vi "aux-builder.parser.vi"(8 "error in":errorcluster, 10 "Proc Name":string, 11 "Flow":T2[](array[typedef])) -> (0 "error out":errorcluster, 3 "Aux Conf out":T1={"Source"="Source ...", "SourceStatus"=FALSE, "Dest"="Auxiliary ...", "DestStatus"=FALSE, "Pulse"=0, "Period"=0, "Proc Name"=""} {"Period" format="Period [s]: %d"; "Pulse" format="Pulse [s]: %d"})   [LabVIEW 2024]
uses:
  controls/UiStepBuilder.ctl
  controls/type.step-builder.ctl
  controls/type.aux.ctl
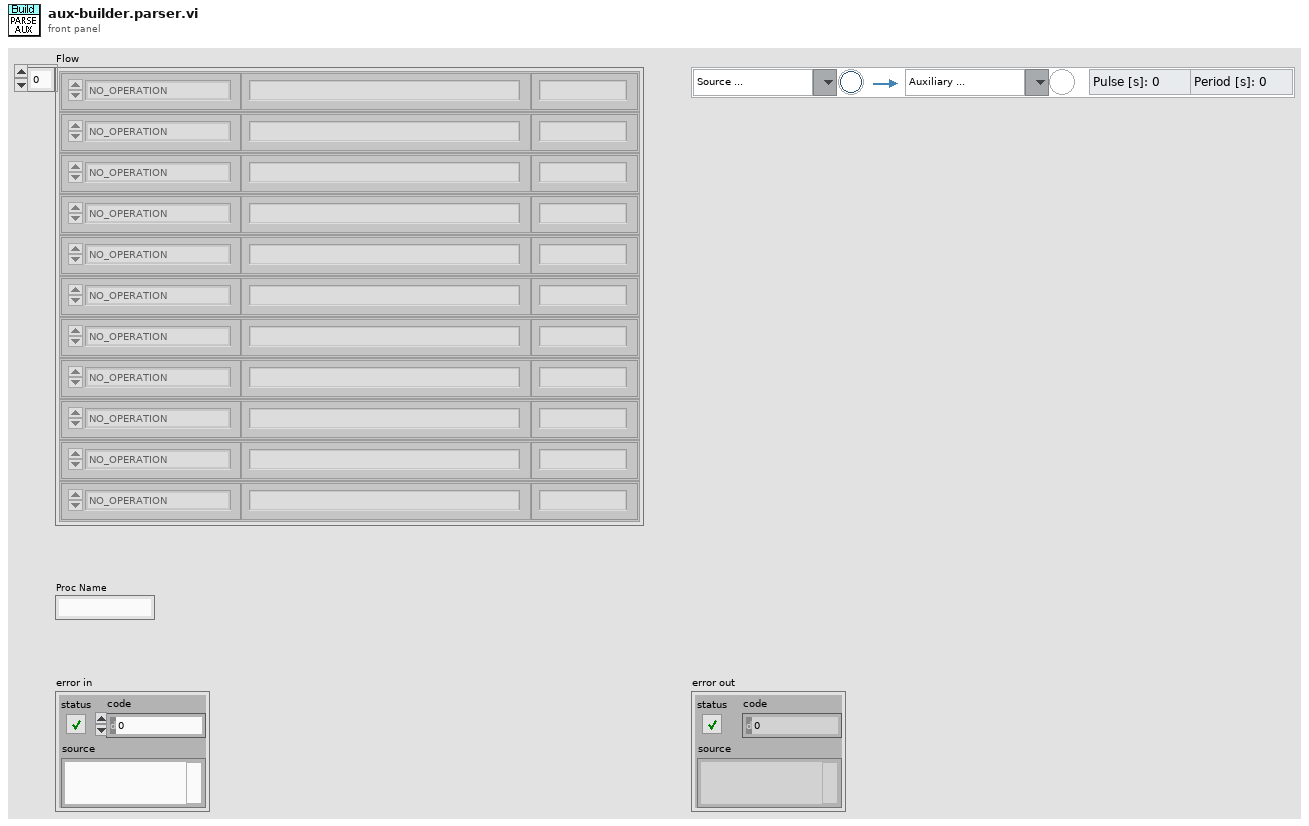
[diagram p1: front panel]
types:
  T1 = typedef "type.aux.ctl" = cluster{"Source":string, "SourceStatus":bool, "Dest":string, "DestStatus":bool, "Pulse":u16, "Period":u16, "Proc Name":string}
  T2 = typedef "UiStepBuilder.ctl" = cluster{"Step Function":T3, "ParamString":string, "Step Label":string}
  T3 = typedef "type.step-builder.ctl" = enum16{"NO_OPERATION", "DELAY-JUMP", "DELAY", "JUMP", "COMPLETE", "SCHEDULER", "IRR-CHECK", "UNIT-CHECK", "UNIT-SAMPLE", "UNIT-DOSE", "LOG-REPORT", "LOG-MESSAGE", "IO-READ", "IO-READ-MANY", "IO-WRITE", "IO-COMPARE-OUT", "IO-COMPARE-IN", "PROC-START", "PROC-STOP", "PROC-LOAD", "PROC-IS-COMPLETED", "RECORD-MOVE", "GET-RH", "GET-UV", "GET-WD", "GET-WS", "OCS-CHECK", "OCS-RECORD"}
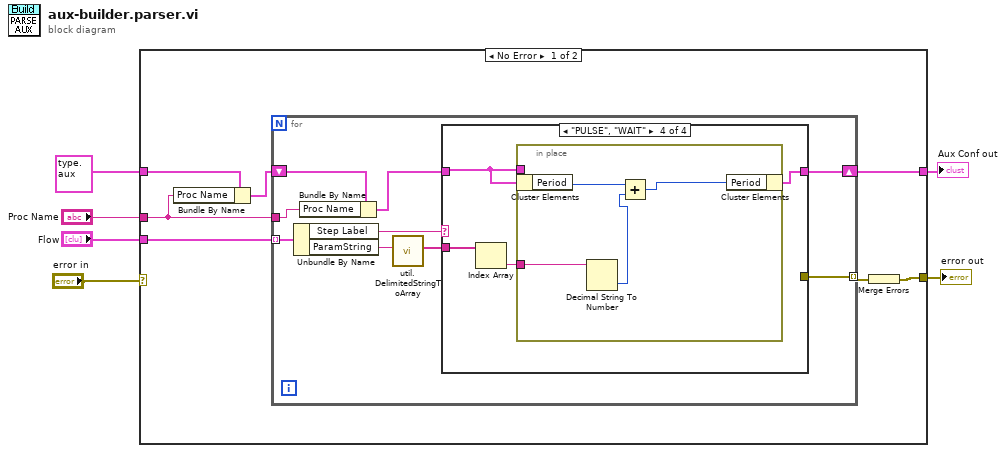
[diagram p0: block diagram]
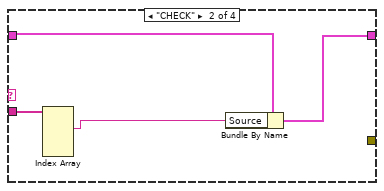
[diagram p3: hidden frame]
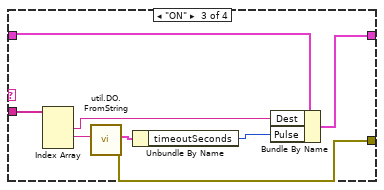
[diagram p4: hidden frame]
diagram:
  n1 = case shown="No Error" "error in" {
    selector: "error in" -> [_ w45]
    tunnel: "Flow" -> [w13 _]
    tunnel: T1 {"Source"="Source ...", "SourceStatus"=FALSE, "Dest"="Auxiliary ...", "DestStatus"=FALSE, "Pulse"=0, "Period"=0, "Proc Name"=""} ("Cluster 2") -> [w12 w44]
    tunnel: [w11 w44] -> w5
    tunnel: [w10 w45] -> w4
    tunnel: "Proc Name" -> [w9 _]
    frame No Error {
      n2 = Bundle By Name(cluster=w12, "Proc Name"=w9) -> (w7:T1)
      n3 = for {
        tunnel: w13 -> [w22] mode=indexing
        shift-right: [w18] -> w11
        shift-left: w7 -> [w15]
        tunnel: [w17] -> w8 mode=indexing
        tunnel: w9 -> [w16]
        n4 = Unbundle By Name(w22) -> ("Step Label"=w21:string, "ParamString"=w20:string)
        n5 = Bundle By Name(cluster=w15, "Proc Name"=w16) -> (w14:T1)
        n6 = call "util.DelimitedStringToArray.vi"("delimitaed string"=w20) -> ("array out"=w19:string[])  [unwired: 10 in]
        n7 = case shown="\"PULSE\", \"WAIT\"" w21 {
          tunnel: w14 -> [w23 w27 w35 w37]
          tunnel: w19 -> [_ w25 w33 w39]
          tunnel: [w23 w26 w34 w36] -> w18
          tunnel: [_ _ w29 _] -> w17
          frame Default {
          }
          frame "CHECK" {
            n8 = Index Array(array=w25) -> (element #1=w24:string)  [unwired: 4 in, 3 out]
            n9 = Bundle By Name(cluster=w27, "Source"=w24) -> (w26:T1)
          }
          frame "ON" {
            n10 = Index Array(array=w33) -> (element #1=w28:string, element #2=w32:string)  [unwired: 3 in, 1 out]
            n11 = call "util.DO.FromString.vi"("initial string"=w32) -> ("error IO"=w29:errorcluster, "output cluster"=w31:cluster{"state":bool, "timeoutSeconds":u16})  [unwired: 9 in]
            n12 = Unbundle By Name(w31) -> ("timeoutSeconds"=w30:u16)
            n13 = Bundle By Name(cluster=w35, "Dest"=w28, "Pulse"=w30) -> (w34:T1)
          }
          frame "PULSE", "WAIT" {
            n14 = Index Array(array=w39) -> (element=w38:string)  [unwired: 1 in]
            n15 = in-place {
              in-place-border: w37 -> [_]
              in-place-border: w38 -> [w43]
              n16 = in-place-cluster #1(w37) -> ("Period"=w42:u16)
              n17 = Decimal String To Number(string=w43) -> (number=w41:i32)  [unwired: 2 in, 1 out]
              n18 = Add(x=w42, y=w41) -> (x+y=w40:i32)
              n19 = in-place-cluster #1("Period"=w40) -> (w36:T1)
            }
          }
        }
      }
      n20 = Merge Errors(w8) -> (w10:errorcluster)
    }
    frame Error {
    }
  }
  "Aux Conf out" <- w5
  "error out" <- w4
